vi "Gen_RND_In_Range.vi"(0 "Upper Bound":dbl, 7 "Lower Bound":dbl) -> (6 "RND_In_Range":dbl)   [LabVIEW 2020]
uses:
  <vilib>/numeric/Random Number (Range) DBL.vi
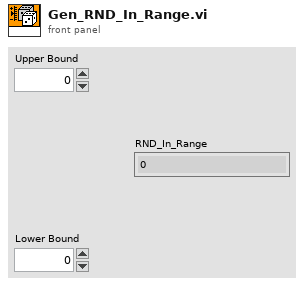
[diagram p1: front panel]
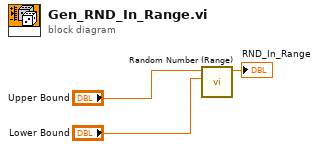
[diagram p0: block diagram]
diagram:
  n1 = call-poly <vilib>:"Random Number (Range).vi"("lower bound (0)"="Lower Bound", "upper bound (100)"="Upper Bound") -> ("number"=→"RND_In_Range":dbl)  [unwired: 9 in]
